vi "Create Session Refnum.vi"(6 "events":T1, 8 "error in (no error)":errorcluster, 10 "abstract":T2, 11 "LIBSSH2_SESSION*":u64 format="%.0x") -> (0 "error out":errorcluster, 3 "session":T3)   [LabVIEW 2017, in "libssh2.lvlib"]
uses:
  libssh2.lvlib
  Session Refnum.ctl
  libssh2_session_abstract.ctl
  lvssh2_session_callback_events.ctl
  lvssh2_session_callback_send_function_input_args_32.ctl
  lvssh2_session_callback_receive_function_input_args_32.ctl
  lvssh2_userauth_keyboard_interactive_response_function_input_args_32.ctl
  lvssh2_session_callback_send_function_input_args_64.ctl
  lvssh2_session_callback_receive_function_input_args_64.ctl
  lvssh2_userauth_keyboard_interactive_response_function_input_args_64.ctl
  Session Refnum Data.ctl
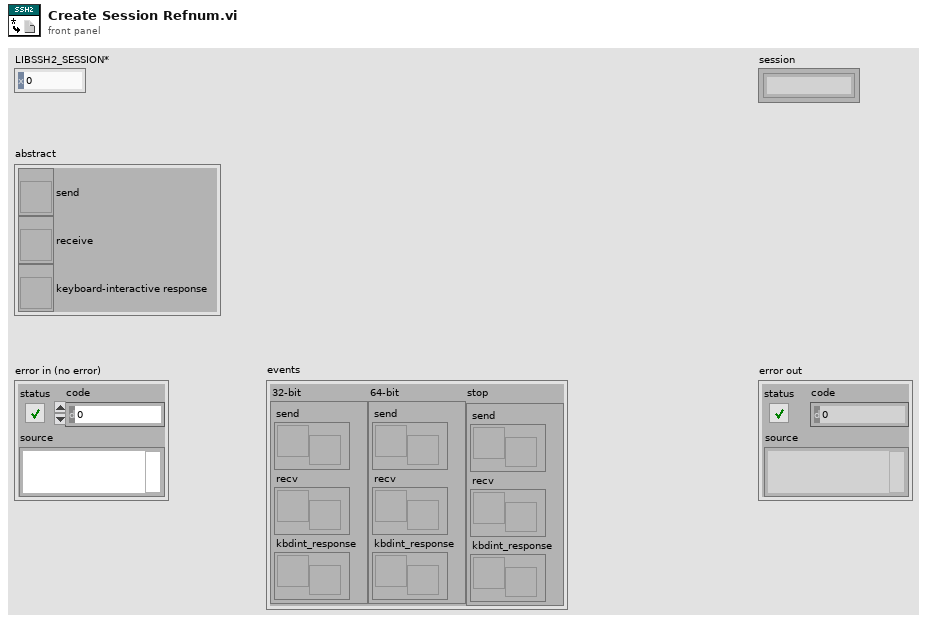
[diagram p1: front panel]
types:
  T1 = typedef "libssh2.lvlib/lvssh2_session_callback_events.ctl" = cluster{"32-bit":cluster{"send":refnum<user-event>, "recv":refnum<user-event>, "kbdint_response":refnum<user-event>}, "64-bit":cluster{"send":refnum<user-event>, "recv":refnum<user-event>, "kbdint_response":refnum<user-event>}, "stop":cluster{"send":refnum<user-event>, "recv":refnum<user-event>, "kbdint_response":refnum<user-event>}}
  T2 = typedef "libssh2.lvlib/libssh2_session_abstract.ctl" = cluster{"send":refnum<vi>, "receive":refnum<vi>, "keyboard-interactive response":refnum<vi>}
  T3 = typedef "libssh2.lvlib/Session Refnum.ctl" = refnum<k1>
  T4 = typedef "libssh2.lvlib/Session Refnum Data.ctl" = cluster{"LIBSSH2_SESSION*":u64, "abstract":T2, "events":T1, "semaphore":T5}
  T5 = typedef "Semaphore RefNum" = refnum<k1>
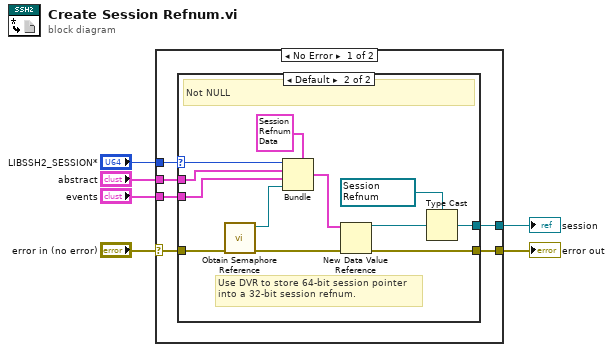
[diagram p0: block diagram]
diagram:
  n1 = case shown="No Error" "error in (no error)" {
    selector: "error in (no error)" -> [w10 w26]
    tunnel: [w12 _] -> w6
    tunnel: "LIBSSH2_SESSION*" -> [w9 _]
    tunnel: [w11 w26] -> w4
    tunnel: "abstract" -> [w8 _]
    tunnel: "events" -> [w7 _]
    frame No Error {
      n2 = case shown="Default" w9 {
        selector: w9 -> [_ w21]
        tunnel: [_ w23] -> w12
        tunnel: [w13 w22] -> w11
        tunnel: w10 -> [w13 w16]
        tunnel: w8 -> [_ w19]
        tunnel: w7 -> [_ w18]
        frame 0 {
          # "NULL"
        }
        frame Default {
          w24 = T3 refnum items=["Session"] ("session")
          # "Use DVR to store 64-bit session pointer\ninto a 32-bit session refnum."
          # "Not NULL"
          n3 = call <vilib>:"Obtain Semaphore Reference.vi"("error in (no error)"=w16) -> ("error out"=w15:errorcluster, "semaphore"=w14:T5)  [unwired: 4 in, 1 out]
          n4 = Bundle(cluster=T4 {"LIBSSH2_SESSION*"=0, "abstract"={"send"=refnum, "receive"=refnum, "keyboard-interactive response"=refnum}, "events"={"32-bit"={"send"=refnum, "recv"=refnum, "kbdint_response"=refnum}, "64-bit"={"send"=refnum, "recv"=refnum, "kbdint_response"=refnum}, "stop"={"send"=refnum, "recv"=refnum, "kbdint_response"=refnum}}, "semaphore"=refnum} ("session data"), "LIBSSH2_SESSION*"=w21, "abstract"=w19, "events"=w18, "semaphore"=w14) -> (w20:T4)
          n5 = New Data Value Reference(data value=w20, error in=w15) -> (data value reference=w25:refnum<data-value>, error out=w22:errorcluster)
          n6 = Type Cast(type=w24, x=w25) -> (*(type *) &x=w23:T3)
        }
      }
    }
    frame Error {
    }
  }
  "session" <- w6
  "error out" <- w4
